vi "create file directory if not found [test].vi"() -> ()   [LabVIEW 2016]
uses:
  file permissions action.ctl
panel:
  out "permissions":i16 format="%o"
  out "error out":errorcluster
  out "created?":bool
  in  "file directory":path=path "C:/Program Files (x86)/National Instruments/RT Images/User Components/C Series Module Detection"
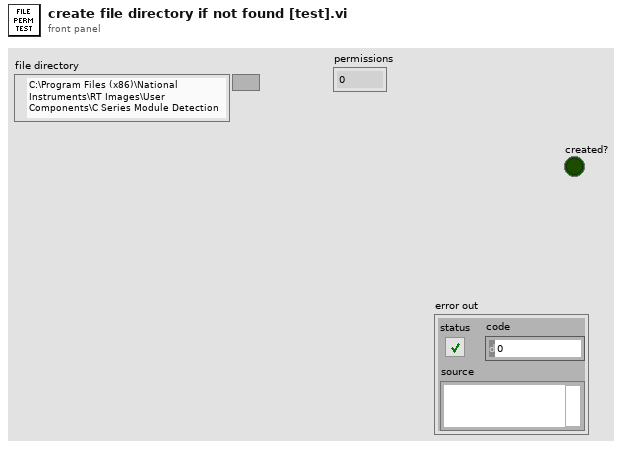
[diagram p1: front panel]
types:
  T1 = typedef "file permissions action.ctl" = enum16{"get", "set", "reset"}
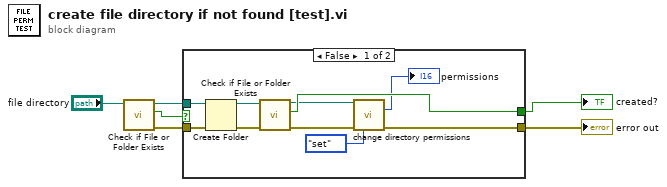
[diagram p0: block diagram]
diagram:
  n1 = call <vilib>:"Check if File or Folder Exists.vi"("path"="file directory") -> ("error out"=w3:errorcluster, "file or folder exists?"=w5:bool, "dup path"=w4:path)  [unwired: 8 in]
  n2 = case shown="False" w5 {
    tunnel: w4 -> [w14 _]
    tunnel: w3 -> [w16 w17]
    tunnel: [w9 w17] -> w1
    tunnel: [w15 _] -> w2
    frame False {
      n3 = Create Folder(path (use dialog)=w14, error in=w16) -> (created path=w13:path, error out=w12:errorcluster)  [unwired: 1 in, 1 out]
      n4 = call <vilib>:"Check if File or Folder Exists.vi"("error in (no error)"=w12, "path"=w13) -> ("error out"=w10:errorcluster, "file or folder exists?"=w15:bool, "dup path"=w8:path)  [unwired: 7 in]
      n5 = call "change directory permissions.vi"("directory"=w8, "error in"=w10, "action (get)"=file_permissions_action."set") -> ("permissions"=→"permissions":i16, "error out"=w9:errorcluster)  [unwired: 10 in, 1 out]
    }
    frame True {
    }
  }
  "created?" <- w2
  "error out" <- w1
